vi "Change Bookmark Filter.vi"(8 "Error In":errorcluster, 10 "Data":variant, 11 "State In":T1) -> (0 "Error Out":errorcluster, 3 "State Out":T1)   [LabVIEW 2017, in "Bookmark Manager.lvlib"]
uses:
  Bookmark Manager.lvlib
  State.ctl
  VI Bookmark.ctl
  VI Information.ctl
  Application Information.ctl
  Bookmarks Views.ctl
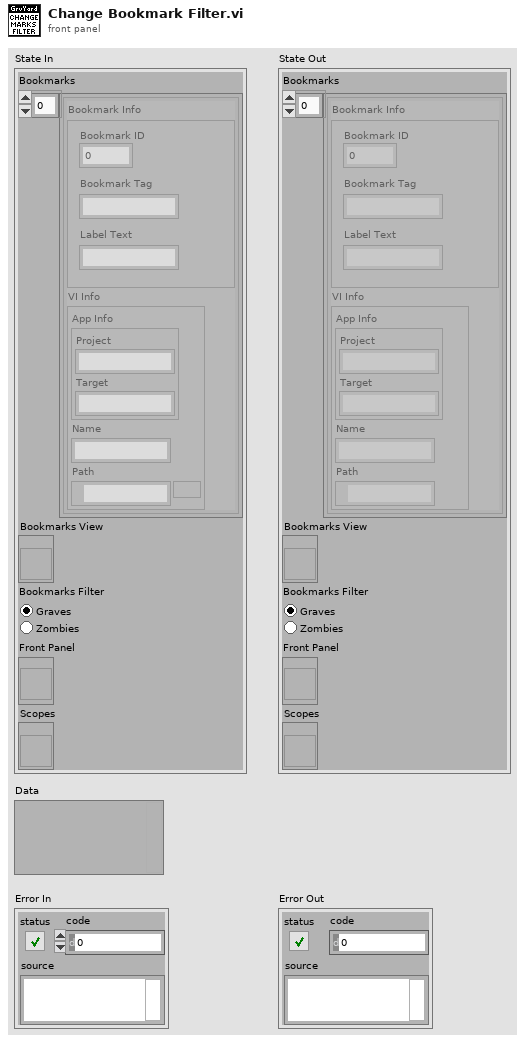
[diagram p1: front panel]
types:
  T1 = typedef "Bookmark Manager.lvlib/State.ctl" = cluster{"Bookmarks":T2[], "Bookmarks View":refnum<vi>, "Bookmarks Filter":T5, "Front Panel":refnum<vi>, "Scopes":refnum<vi>}
  T2 = typedef "Bookmark Manager.lvlib/VI Bookmark.ctl" = cluster{"Bookmark Info":cluster{"Bookmark ID":u32, "Bookmark Tag":string, "Label Text":string}, "VI Info":T3}
  T3 = typedef "Bookmark Manager.lvlib/VI Information.ctl" = cluster{"App Info":T4, "Name":string, "Path":path}
  T4 = typedef "Bookmark Manager.lvlib/Application Information.ctl" = cluster{"Project":string, "Target":string}
  T5 = typedef "Bookmark Manager.lvlib/Bookmarks Views.ctl" = enum32{"Graves", "Zombies"}
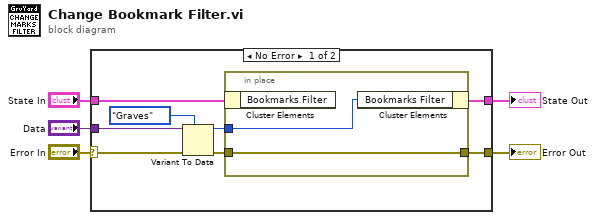
[diagram p0: block diagram]
diagram:
  n1 = case shown="No Error" "Error In" {
    selector: "Error In" -> [w8 w16]
    tunnel: [w11 w17] -> w5
    tunnel: "State In" -> [w10 w17]
    tunnel: "Data" -> [w9 _]
    tunnel: [w6 w16] -> w2
    frame No Error {
      n2 = Variant To Data(error in=w8, type=Bookmarks_Views."Graves" ("Bookmarks Type"), Variant=w9) -> (data=w12:T5, error out=w7:errorcluster)
      n3 = in-place {
        in-place-border: w12 -> [w14]
        in-place-border: w7 -> [w15]
        in-place-border: [w15] -> w6
        n4 = in-place-cluster #1(w10) -> ()  [unwired: 1 out]
        n5 = in-place-cluster #1("Bookmarks Filter"=w14) -> (w11:T1)
      }
    }
    frame Error {
    }
  }
  "State Out" <- w5
  "Error Out" <- w2
